vi "Calculate Required Steering Angle.vi"(7 "constraint error tolerance (1E-12)":dbl=1e-12, 8 "error in (no error)":errorcluster, 9 "wheel frame velocity":dbl[](array[numeric]), 11 "fixed wheel in":refnum<class "NI_Robotics_Fixed Wheel.lvclass">) -> (0 "error out":errorcluster, 2 "required steering angle (rad)":dbl, 3 "fixed wheel out":refnum<class "NI_Robotics_Fixed Wheel.lvclass">)   [LabVIEW 2017, in "NI_Robotics_Fixed Wheel.lvclass"]
uses:
  <vilib>/robotics/Steering/Fixed Wheel/NI_Robotics_Fixed Wheel.lvclass
  c:/Program Files (x86)/National Instruments/LabVIEW 2017/vi.lib/robotics/Steering/Wheel/NI_Robotics_Wheel.lvclass
  <vilib>/robotics/Steering/Wheel/NI_Robotics_Wheel.lvclass/NI_Robotics_Wheel.ctl
  <vilib>/robotics/Utilities/NI_Robotics Utilities.lvlib
  <vilib>/robotics/Steering/Wheel/NI_Robotics_Wheel.lvclass
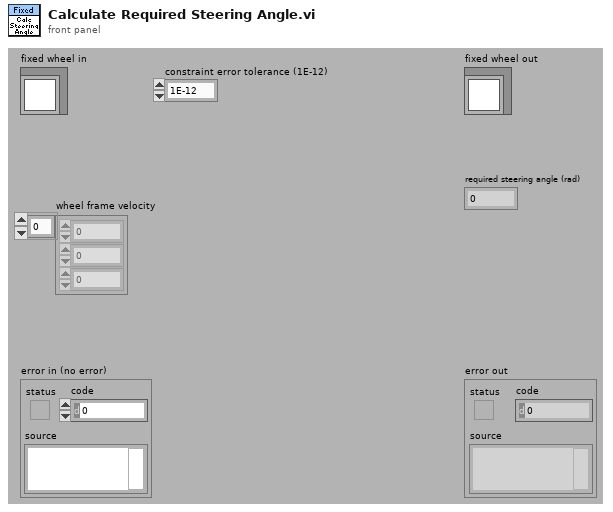
[diagram p1: front panel]
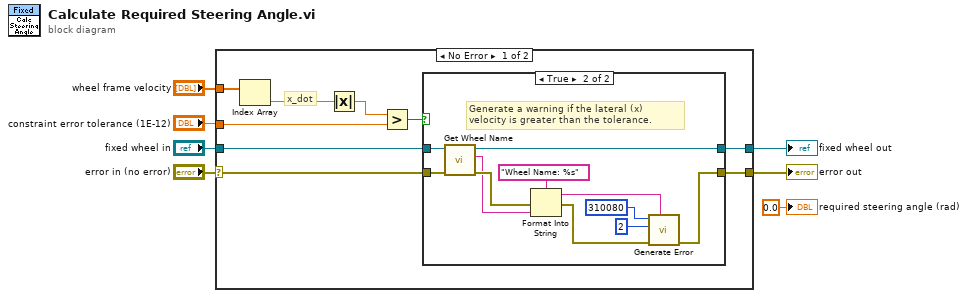
[diagram p0: block diagram]
diagram:
  n1 = case shown="No Error" "error in (no error)" {
    selector: "error in (no error)" -> [w11 w30]
    tunnel: "fixed wheel in" -> [w12 w31]
    tunnel: [w14 w31] -> w5
    tunnel: "wheel frame velocity" -> [w10 _]
    tunnel: [w13 w30] -> w2
    tunnel: "constraint error tolerance (1E-12)" -> [w16 _]
    frame No Error {
      # "x_dot"
      n2 = Index Array(array=w10) -> (element=w9:dbl)  [unwired: 1 in]
      n3 = Absolute Value(x=w9) -> (abs(x)=w8:dbl)
      n4 = Greater?(x=w8, y=w16) -> (0:w15:bool)
      n5 = case shown="True" w15 {
        tunnel: w12 -> [w18 w26]
        tunnel: w11 -> [w17 w24]
        tunnel: [w18 w25] -> w14
        tunnel: [w17 w28] -> w13
        frame False {
        }
        frame True {
          # "Generate a warning if the lateral (x) velocity is greater than the tolerance."
          n6 = call <vilib>:"Get Wheel Name.vi"("error in (no error)"=w24, "wheel in"=w26) -> ("error out"=w23:errorcluster, "wheel name"=w21:string, "wheel out"=w25:refnum<class "NI_Robotics_Fixed Wheel.lvclass">)  [unwired: 7 in]
          n7 = Format Into String(format string="Wheel Name: %s", error in=w23, w21) -> (resulting string=w19:string, error out=w22:errorcluster)  [unwired: 1 in]
          n8 = call <vilib>:"Generate Error.vi"("<append> (\"\")"=w19, "error in (no error)"=w22, "chain levels to remove (1)"=2, "code"=310080) -> ("error out"=w28:errorcluster)  [unwired: 7 in]
        }
      }
    }
    frame Error {
    }
  }
  "error out" <- w2
  "fixed wheel out" <- w5
  "required steering angle (rad)" <- 0.0 ("Required Steering Angle")
